vi "Add Response RTM.vi"(8 "error in (no error)":errorcluster, 11 "Node Ptr":u64 format="%.0x") -> (0 "error out":errorcluster)   [LabVIEW 2018, in "Instrument Addon System Explorer.lvlib"]
uses:
  Instrument Addon System Explorer.lvlib
  APIs/Scripting API/TypeDefs/Wait Response Settings.ctl
  APIs/Scripting API/TypeDefs/Linked Channel.ctl
  <vilib>/NI Veristand/Custom Device API/Custom Device Item Ref.ctl
  APIs/Scripting API/Messages/Add Response - Wait (sec).vi
  APIs/Scripting API/Instrument Addon Scripting API.lvlib
  <vilib>/NI Veristand/Custom Device API/Custom Device API.lvlib
panel:
  in  "Tag":string
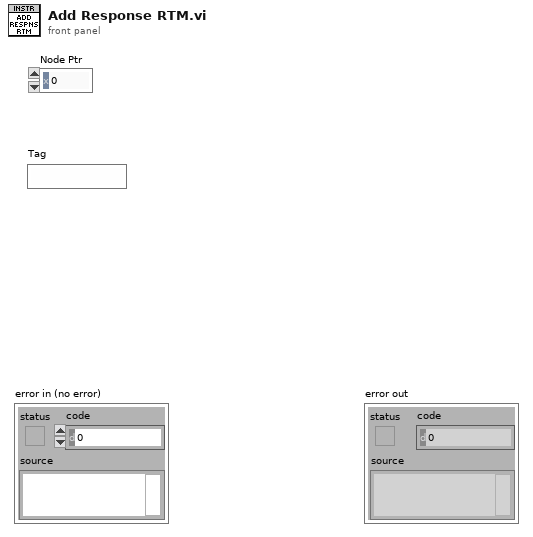
[diagram p1: front panel]
types:
  T1 = typedef "Instrument Addon Scripting API.lvlib/Wait Response Settings.ctl" = cluster{"Response Format":string, "Linked Channels":T2[], "Wait value (sec)":dbl, "Use Wait Channel":bool, "Channel Refnum":T3}
  T2 = typedef "Instrument Addon Scripting API.lvlib/Linked Channel.ctl" = cluster{"Variable Name":string, "Channel Refnum":T3}
  T3 = typedef "Custom Device API.lvlib/Custom Device Item Ref.ctl" = u64
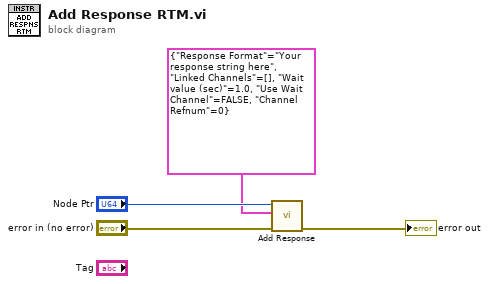
[diagram p0: block diagram]
diagram:
  n1 = call-poly "Add Response.vi"("error in (no error)"="error in (no error)", "Settings"=T1 {"Response Format"="Your response string here", "Linked Channels"=[], "Wait value (sec)"=1.0, "Use Wait Channel"=FALSE, "Channel Refnum"=0}, "Message in"="Node Ptr") -> ("error out"=→"error out":errorcluster)  [unwired: 7 in, 1 out]
